vi "加载控件.vi"(8 "error in (no error)":errorcluster caption="错误输入（无错误）", 11 "程序 输入":refnum<class "程序.lvclass">) -> (0 "error out":errorcluster caption="错误输出", 3 "程序 输出":refnum<class "程序.lvclass">)   [LabVIEW 2020, in "程序.lvclass"]
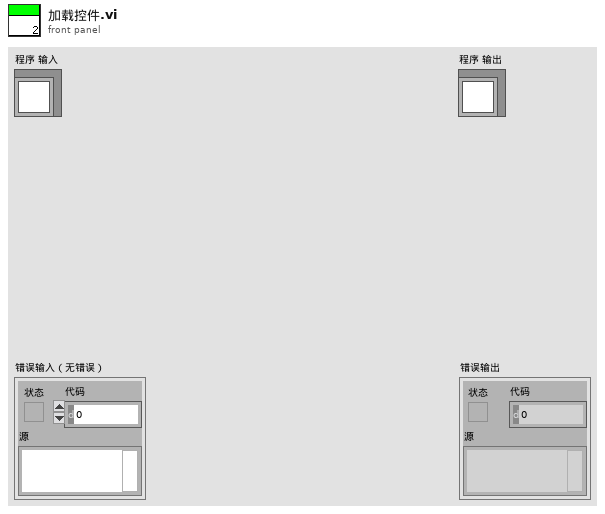
[diagram p1: front panel]
types:
  T1 = typedef "imagedata.ctl" = cluster{"image type":i32, "image depth":i32, "image":u8[], "mask":u8[], "colors":u32[], "Rectangle":cluster{"left":i16, "top":i16, "right":i16, "bottom":i16}}
  T2 = cluster{"new picture":picture, string, string, string, "image data":T1}
  T3 = cluster{"new picture":picture, string, string, string, "image data":T1}[]
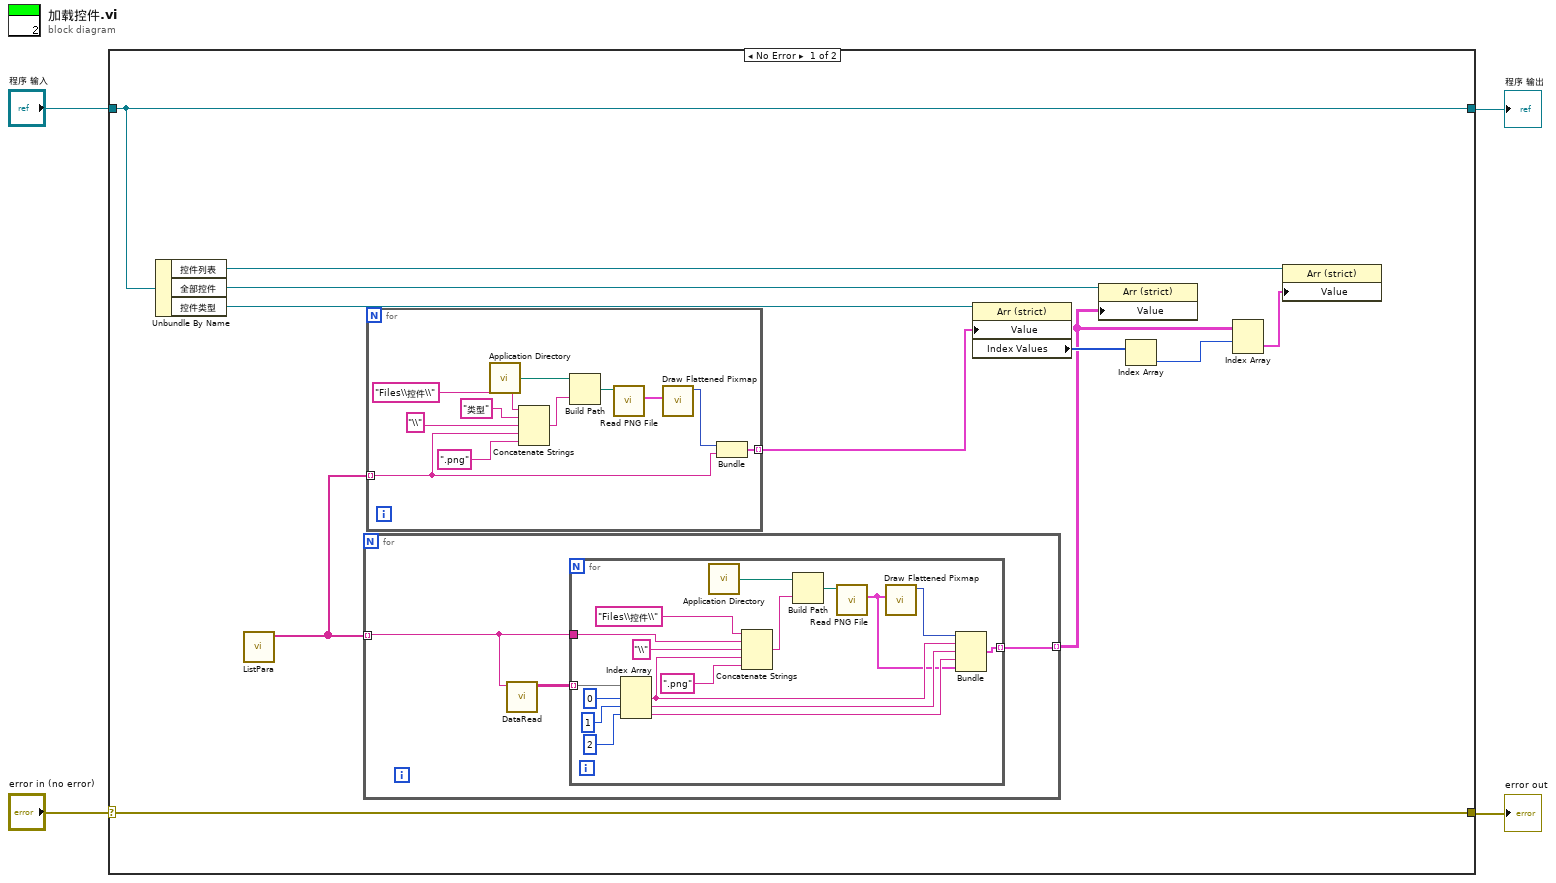
[diagram p0: block diagram]
diagram:
  n1 = case shown="No Error" "error in (no error)" {
    selector: "error in (no error)" -> [w15 w48]
    tunnel: [w15 w48] -> w3
    tunnel: [w14 w47] -> w1
    tunnel: "程序 输入" -> [w14 w47]
    frame No Error {
      n2 = Unbundle By Name(w14) -> ("控件列表"=w9:refnum<vi>, "全部控件"=w13:refnum<vi>, "控件类型"=w11:refnum<vi>)
      n3 = call "ListPara.vi"() -> ("Paras"=w12:string[])  [unwired: 11 in]
      n4 = for {
        tunnel: w12 -> [w27] mode=indexing
        tunnel: [w28] -> w5 mode=indexing
        n5 = call "DataRead.vi"("段名"=w27) -> ("数据"=w29:string[][])  [unwired: 10 in]
        n6 = for {
          tunnel: w29 -> [w39] mode=indexing
          tunnel: [w40] -> w28 mode=indexing
          tunnel: w27 -> [w31]
          n7 = Index Array(array=w39, index #1=0 ("索引"), index #2=1 ("索引"), index #3=2 ("索引")) -> (element #1=w38:string, element #2=w35:string, element #3=w33:string)
          n8 = call <vilib>:"Application Directory.vi"() -> ("Application Directory"=w46:path)
          n9 = Concatenate Strings("Files\\控件\\" ("名称或相对路径"), w31, "\\" ("字符串"), w38, ".png" ("字符串")) -> (w44:string)
          n10 = Build Path(base path=w46, name or relative path=w44) -> (appended path=w42:path)
          n11 = call <vilib>:"Read PNG File.vi"("path to PNG file"=w42) -> ("image data"=w30:T1)  [unwired: 8 in, 2 out]
          n12 = call <vilib>:"Draw Flattened Pixmap.vi"("image data"=w30) -> ("new picture"=w41:picture)  [unwired: 8 in]
          n13 = Bundle("new picture"=w41, w38, w35, w33, "image data"=w30) -> (w40:T2)  [unwired: 1 in]
        }
      }
      n14 = for {
        tunnel: w12 -> [w17] mode=indexing
        tunnel: [w16] -> w10 mode=indexing
        n15 = call <vilib>:"Application Directory.vi"() -> ("Application Directory"=w20:path)
        n16 = Concatenate Strings("Files\\控件\\" ("名称或相对路径"), "类型" ("字符串"), "\\" ("字符串"), w17, ".png" ("字符串")) -> (w22:string)
        n17 = Build Path(base path=w20, name or relative path=w22) -> (appended path=w24:path)
        n18 = call <vilib>:"Read PNG File.vi"("path to PNG file"=w24) -> ("image data"=w25:T1)  [unwired: 8 in, 2 out]
        n19 = call <vilib>:"Draw Flattened Pixmap.vi"("image data"=w25) -> ("new picture"=w18:picture)  [unwired: 8 in]
        n20 = Bundle("new picture"=w18, "String"=w17) -> (w16:cluster{"new picture":picture, "String":string})  [unwired: 1 in]
      }
      n21 = property class="Arr (strict)"(reference=w11, "Value"=w10) -> ("Index Values"=w7:u32[])  [unwired: 1 in, 2 out]
      n22 = property class="Arr (strict)"(reference=w13, "Value"=w5) -> ()  [unwired: 1 in, 2 out]
      n23 = Index Array(array=w7) -> (element=w6:u32)  [unwired: 1 in]
      n24 = Index Array(array=w5, index (row)=w6) -> (element=w8:T3)  [unwired: 1 in]
      n25 = property class="Arr (strict)"(reference=w9, "Value"=w8) -> ()  [unwired: 1 in, 2 out]
    }
    frame Error {
    }
  }
  "error out" <- w3
  "程序 输出" <- w1
